vi "WFGenerateA.vi"(0 "Sound Type":T2, 1 "Param 0":dbl, 2 "Param 1":dbl, 3 "Param 2":dbl, 4 "Param 3":dbl, 5 "error in (no error)":errorcluster, 8 "WFParameters":T3={"Fs (Hz)"=20000.0, "Amp (V)"=5.0, "Ramp (s)"=0.005, "Dur (s)"=0.25} {"Dur (s)" min=0.0 format="%#_4g"; "Ramp (s)" min=0.0; "Fs (Hz)" min=0.0}, 10 "WFRepetitions":T1={"Del (s)"=0.0, "Int (s)"=0.0, "N"=1} {"Int (s)" min=0.0 format="%#_4g"; "Del (s)" min=0.0 format="%#_4f"}) -> (14 "Waveform Out":waveform(dbl), 19 "error out":errorcluster)   [LabVIEW 2013]
uses:
  WFParameters.ctl
  WFTypes.ctl
  WFRepetitions.ctl
panel:
  out "Waveform Graph":waveform(dbl)(graph)
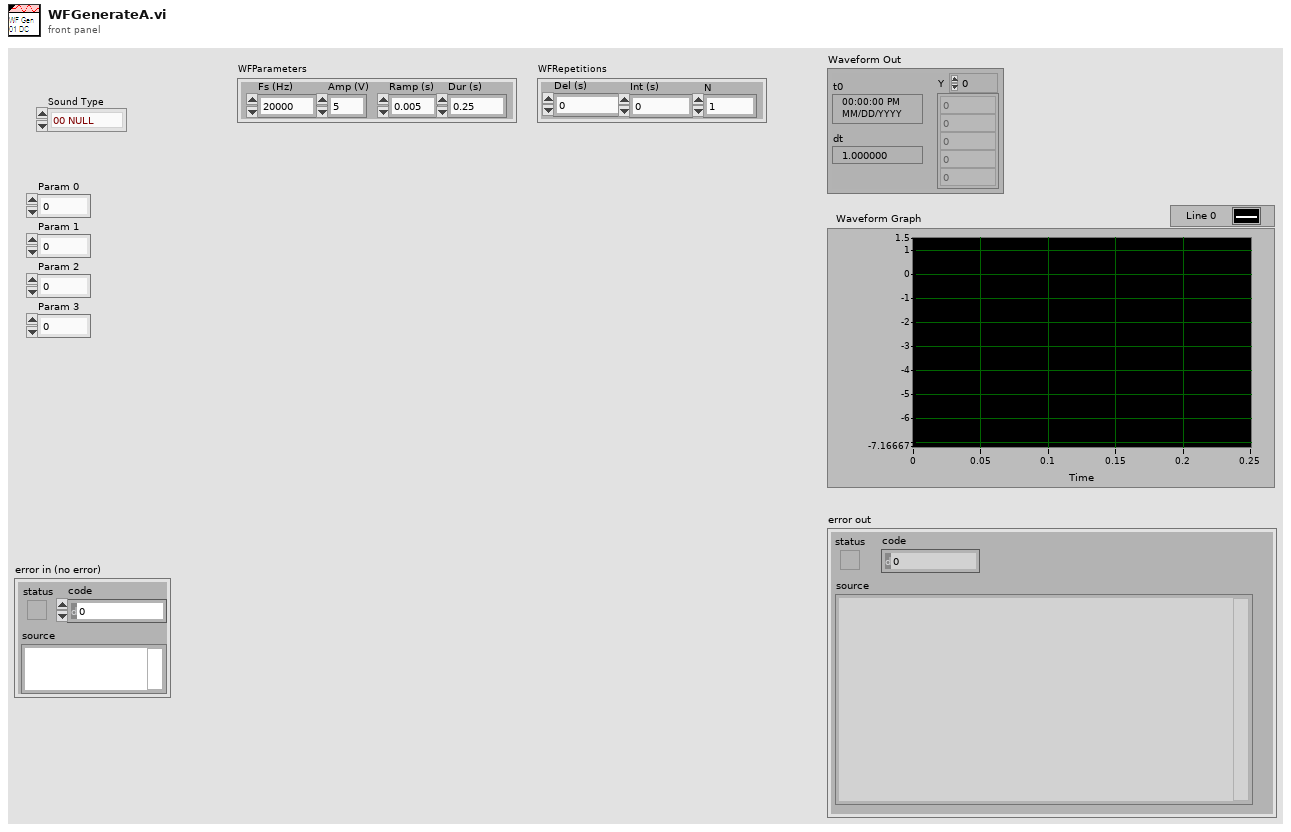
[diagram p1: front panel]
types:
  T1 = typedef "WFRepetitions.ctl" = cluster{"Del (s)":dbl, "Int (s)":dbl, "N":i32}
  T2 = typedef "WFTypes.ctl" = enum16{"00 NULL", "01 DC", "02 Noise", "03 Pure Tone", "04 FM Sweep"}
  T3 = typedef "WFParameters.ctl" = cluster{"Fs (Hz)":dbl, "Amp (V)":dbl, "Ramp (s)":dbl, "Dur (s)":dbl}
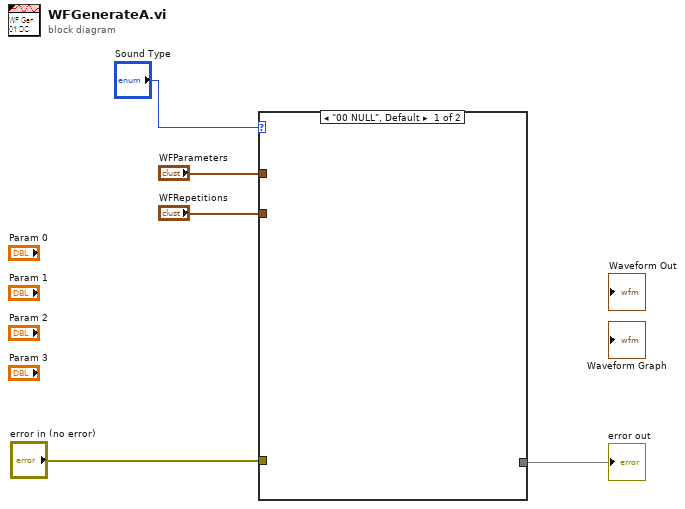
[diagram p0: block diagram]
diagram:
  n1 = case shown="\"00 NULL\", Default" "Sound Type" {
    tunnel: "WFParameters" -> [_ _]
    tunnel: "WFRepetitions" -> [_ _]
    tunnel: "error in (no error)" -> [_ _]
    tunnel: [_ _] -> w1
    frame "00 NULL", Default {
    }
    frame "01 DC" {
    }
  }
  "error out" <- w1
